vi "Save.vi"(8 "error in (no error)":errorcluster, 10 "Save":bool, 11 "Top Level in":refnum<class "Top Level.lvclass">) -> (0 "error out":errorcluster, 3 "Top Level out":refnum<class "Top Level.lvclass">)   [LabVIEW 2021, in "Top Level.lvlib" / "Top Level.lvclass"]
uses:
  Top Level.lvclass
  Top Level.lvclass/Top Level.ctl
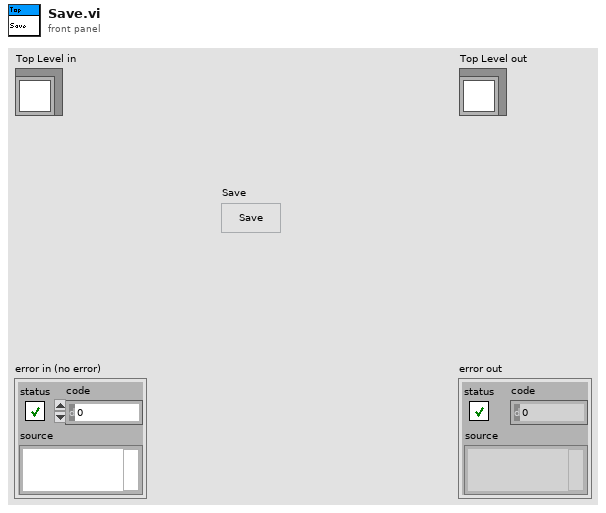
[diagram p1: front panel]
types:
  T1 = enum16{"open", "replace", "create", "open or create", "replace or create", "replace or create with confirmation"}
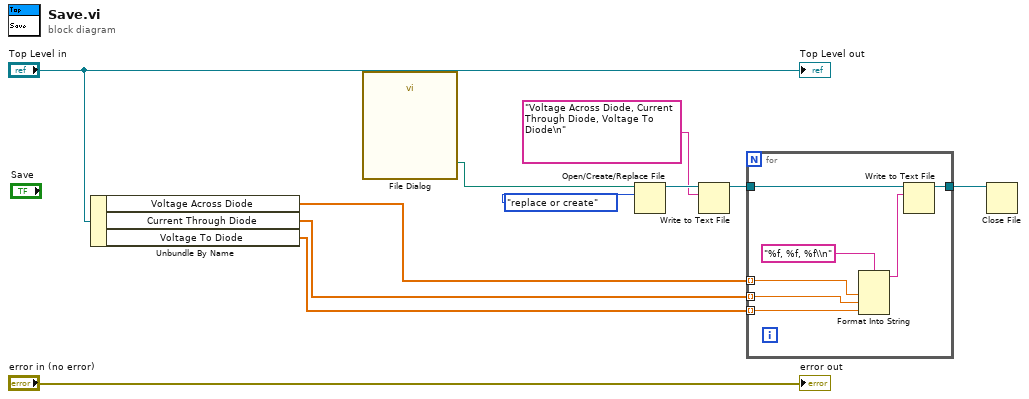
[diagram p0: block diagram]
diagram:
  n1 = Unbundle By Name("Top Level in") -> ("Voltage Across Diode"=w6:dbl[], "Current Through Diode"=w5:dbl[], "Voltage To Diode"=w4:dbl[])
  n2 = call "File Dialog"() -> ("selected path"=w1:path)  [unwired: 12 in, 3 out]
  n3 = Open/Create/Replace File(file path (use dialog)=w1, operation (0:open)=T1."replace or create") -> (refnum out=w9:refnum<file>)  [unwired: 4 in, 2 out]
  n4 = Write to Text File(file (use dialog)=w9, text="Voltage Across Diode, Current Through Diode, Voltage To Diode\n") -> (refnum out=w3:refnum<file>)  [unwired: 2 in, 2 out]
  n5 = for {
    tunnel: w6 -> [w18] mode=indexing
    tunnel: w5 -> [w17] mode=indexing
    tunnel: w4 -> [w16] mode=indexing
    tunnel: w3 -> [w15]
    tunnel: [w14] -> w2
    n6 = Format Into String(format string="%f, %f, %f\\n", w18, w17, w16) -> (resulting string=w13:string)  [unwired: 2 in, 1 out]
    n7 = Write to Text File(file (use dialog)=w15, text=w13) -> (refnum out=w14:refnum<file>)  [unwired: 2 in, 2 out]
  }
  n8 = Close File(refnum=w2) -> ()  [unwired: 1 in, 2 out]
  "error out" <- "error in (no error)"
  "Top Level out" <- "Top Level in"
